vi "Hella BLDC CAN read.vi"(8 "Error In":errorcluster, 9 "Expected":u8 format="%.0x", 10 "Index":i32, 11 "Ref In":refnum<k20>) -> (0 "Error Out":errorcluster, 1 "Valid?":bool, 2 "payload":u8[](array[numeric]), 3 "Ref Out":refnum<k20>)   [LabVIEW 2019]
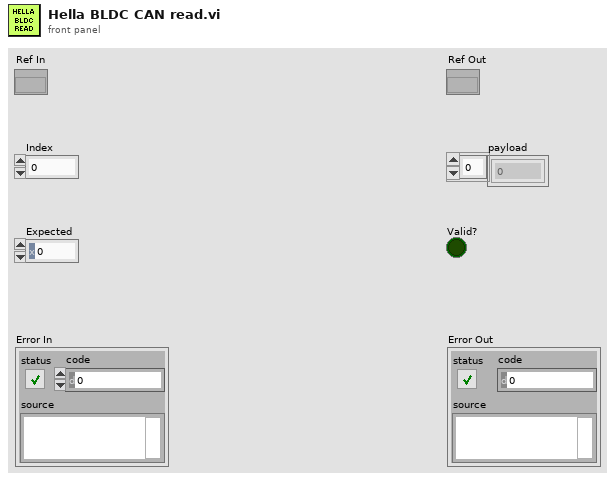
[diagram p1: front panel]
types:
  T1 = typedef "CANFrameControl.ctl" = cluster{"identifier":u32, "extended?":bool, "type":u8, "payload":u8[]}
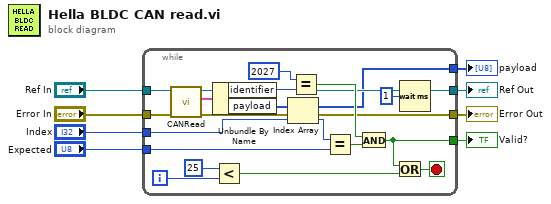
[diagram p0: block diagram]
diagram:
  n1 = while {
    tunnel: "Ref In" -> [w27]
    tunnel: "Error In" -> [w26]
    tunnel: "Index" -> [w23]
    tunnel: "Expected" -> [w19]
    tunnel: [w12] -> w6
    tunnel: [w11] -> w3
    tunnel: [w10] -> w2
    tunnel: [w9] -> w1
    i -> [w16]
    stop <- w14 stop-if-true
    n2 = call <vilib>:"CANRead.vi"("error in (no error)"=w26, "interface object in"=w27) -> ("error out"=w12:errorcluster, "CAN frame"=w24:T1, "interface object out"=w11:refnum<k20>)  [unwired: 6 in, 1 out]
    n3 = Unbundle By Name(w24) -> ("identifier"=w22:u32, "payload"=w10:u8[])
    n4 = Less?(x=25, y=w16) -> (x < y?=w13:bool)
    n5 = Index Array(array=w10, index=w23) -> (element=w20:u8)
    n6 = Equal?(x=u32 2027, y=w22) -> (x = y?=w17:bool)
    n7 = Equal?(x=w20, y=w19) -> (x = y?=w18:bool)
    n8 = And(x=w17, y=w18) -> (x .and. y?=w9:bool)
    n9 = Or(x=w9, y=w13) -> (x .or. y?=w14:bool)
    n10 = Wait (ms)(milliseconds to wait=u32 1) -> ()  [unwired: 1 out]
  }
  "Valid?" <- w1
  "Error Out" <- w6
  "Ref Out" <- w3
  "payload" <- w2
